vi "Load Test Channel.vi"(8 "error in (no error)":errorcluster, 11 "Edit Test Channel Model in":refnum<class "Edit Test Channel Model.lvclass">) -> (0 "error out":errorcluster, 3 "Edit Test Channel Model out":refnum<class "Edit Test Channel Model.lvclass">)   [LabVIEW 2013, in "Edit Test Channel Model.lvlib" / "Edit Test Channel Model.lvclass"]
uses:
  Edit Test Channel Model.lvclass
  Edit Test Channel Model.lvclass/Edit Test Channel Model.ctl
  Common/File IO/File IO.lvlib
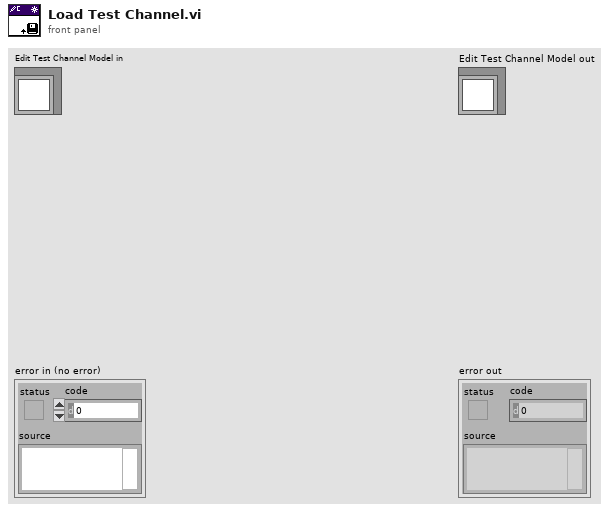
[diagram p1: front panel]
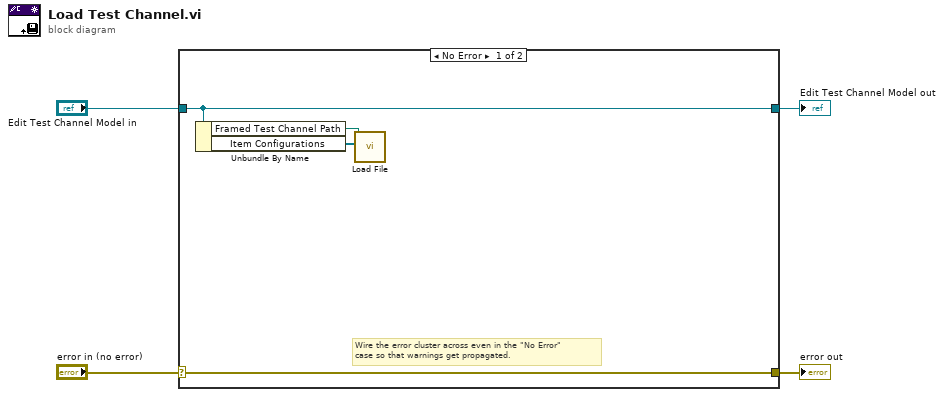
[diagram p0: block diagram]
diagram:
  n1 = case shown="No Error" "error in (no error)" {
    selector: "error in (no error)" -> [w8 w10]
    tunnel: [w8 w10] -> w3
    tunnel: [w6 w9] -> w1
    tunnel: "Edit Test Channel Model in" -> [w6 w9]
    frame No Error {
      # "Wire the error cluster across even in the \"No Error\"\ncase so that warnings get propagated."
      n2 = Unbundle By Name(w6) -> ("Framed Test Channel Path"=w5:path, "Item Configurations"=w7:refnum<class "Item Configuration.lvclass">[])
      n3 = call "Load File.vi"("Item Configurations"=w7, "File Path"=w5) -> ()  [unwired: 9 in, 1 out]
    }
    frame Error {
    }
  }
  "error out" <- w3
  "Edit Test Channel Model out" <- w1
